vi "Error Proc.vi"(8 "error in (no error)":errorcluster, 11 "View Model":T1) -> (0 "error out":errorcluster)   [LabVIEW 2017]
doc: "Serves for different processing available error types."
uses:
  View Model/Controls/View Model.ctl
  View Model/Controls/Shared Model.ctl
  Controls/Error Model.ctl
  Controls/Error Event.ctl
  Controls/Error Type.ctl
  Controller/Controls/Controller Model.ctl
  Controller/Controls/Controller Event.ctl
  Controller/Controls/Controller Command.ctl
  Controller/Controls/Controller Overhead.ctl
  Real-Time/RT Status.ctl
  Real-Time/RT Loop Status.ctl
  Controller/Controls/Controller NStream.ctl
  Controller/Controls/Controller DAQ Data.ctl
  TDMS Logger/Controls/TDMS Model.ctl
  TDMS Logger/Controls/TDMS Event.ctl
  TDMS Logger/Controls/TDMS Command.ctl
  TDMS Logger/Controls/TDMS Overhead.ctl
  TDMS Logger/Controls/TDMS ChanNames.ctl
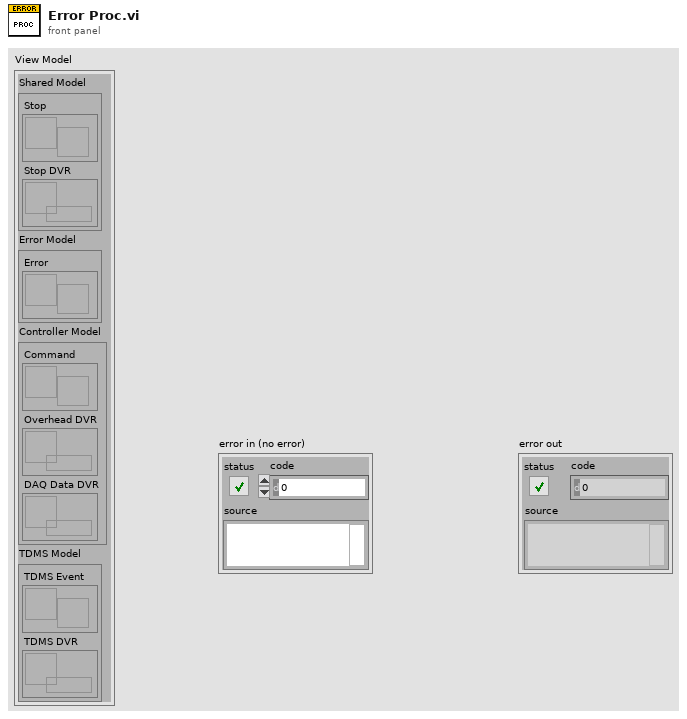
[diagram p1: front panel]
types:
  T1 = typedef "View Model.ctl" = cluster{"Shared Model":T2, "Error Model":T3, "Controller Model":T4, "TDMS Model":T5}
  T2 = typedef "Shared Model.ctl" = cluster{"Stop":refnum<user-event>, "Stop DVR":refnum<data-value>}
  T3 = typedef "Error Model.ctl" = cluster{"Error":refnum<user-event>}
  T4 = typedef "Controller Model.ctl" = cluster{"Command":refnum<user-event>, "Overhead DVR":refnum<data-value>, "DAQ Data DVR":refnum<data-value>}
  T5 = typedef "TDMS Model.ctl" = cluster{"TDMS Event":refnum<user-event>, "TDMS DVR":refnum<data-value>}
  T6 = typedef "Error Type.ctl" = enum16{"Minor", "Critical"}
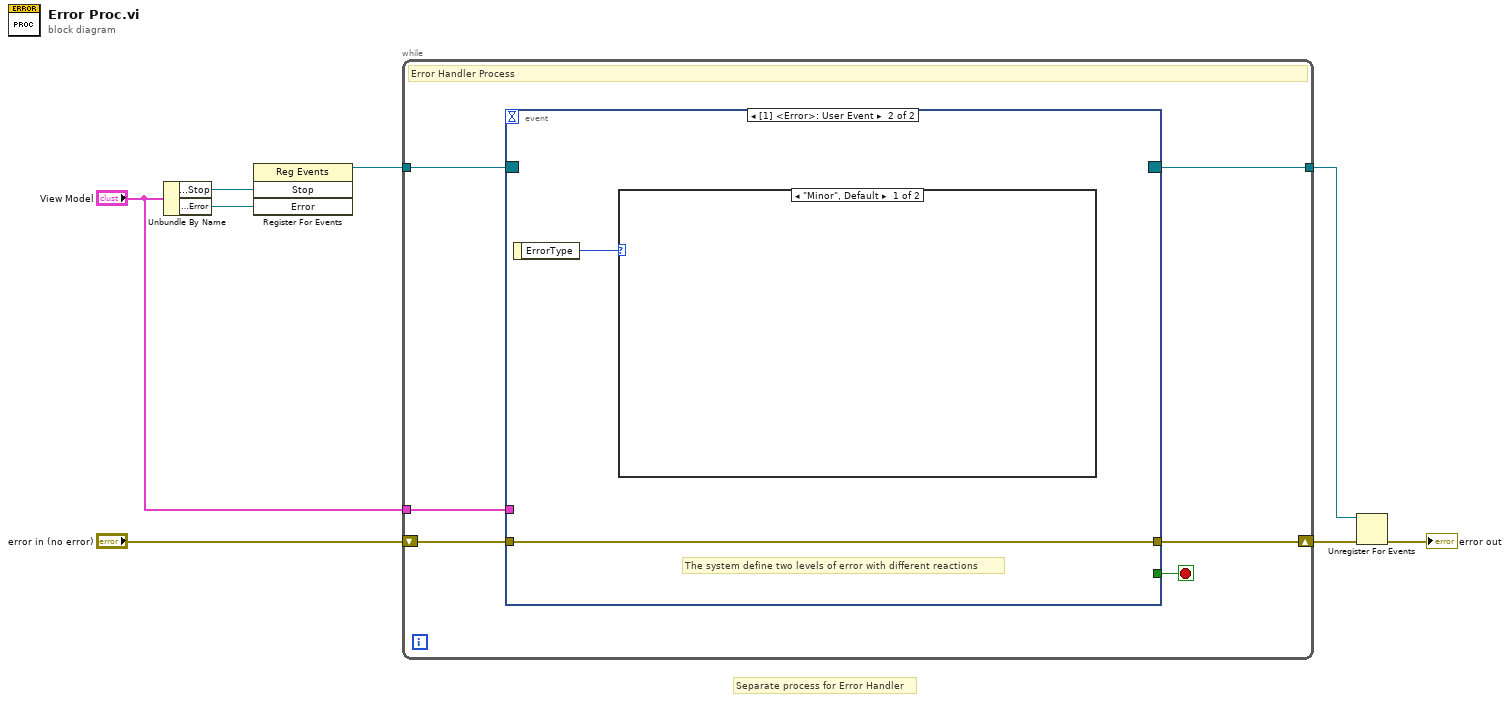
[diagram p0: block diagram]
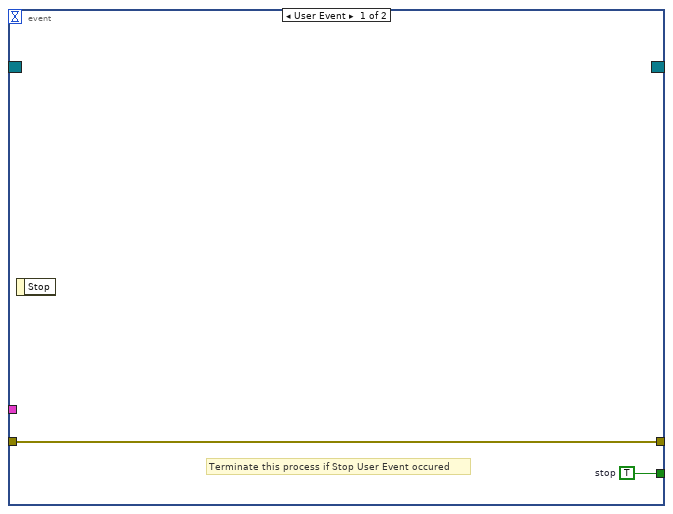
[diagram p2: hidden frame]
diagram:
  # "Separate process for Error Handler"
  n1 = Unbundle By Name("View Model") -> ("Shared Model.Stop"=w8:refnum<user-event>, "Error Model.Error"=w1:refnum<user-event>)
  n2 = register-events(w8, w1) -> (reference out=w7:refnum<event-registration>)  [unwired: 2 in, 1 out]
  n3 = while {
    tunnel: w7 -> [w13]
    shift-right: [w9] -> w4
    shift-left: "error in (no error)" -> [w14]
    tunnel: "View Model" -> [w10]
    tunnel: [w12] -> w3
    stop <- w11 stop-if-true
    # "Error Handler Process"
    n4 = event shown="[1] <Error>: User Event" {
      selector: w13 -> [_ _]
      dyn-events: [_ _] -> w12
      timeout: _ -> [_ _]
      tunnel: w14 -> [w16 w17]
      tunnel: w10 -> [_ _]
      tunnel: [w16 w17] -> w9
      tunnel: [w15 _] -> w11
      event User Event {
        w15 = TRUE  # stop
        # "Terminate this process if Stop User Event occured"
        n5 = event-data() -> ()  [unwired: 1 in, 1 out]
      }
      event User Event {
        # "The system define two levels of error with different reactions"
        n6 = event-data() -> ("ErrorType"=w18:T6)  [unwired: 1 in]
        n7 = case shown="\"Minor\", Default" w18 {
          frame "Minor", Default {
          }
          frame "Critical" {
          }
        }
      }
    }
  }
  n8 = Unregister For Events(event registration refnum=w3, error in=w4) -> (error out=→"error out":errorcluster)
